vi "Load one I16bit Image with metadata from Tiff Stack file.vi"(7 "path to TIFF file":path=path "/HD1/Users/herbertlooser/Desktop/LadungssprŸher.tif", 8 "error in":errorcluster, 10 "Index of image\n to read":i32, 11 "I16 Image":T1) -> (0 "error out":errorcluster, 3 "I16 Image dup":T1)   [LabVIEW 2013, in "Tiff reader.lvlib"]
doc: "This .vi is taken from an online tiff reader. It is able to read 32-bit floating point .tiff images."
uses:
  Tiff reader.lvlib
  <vilib>/vision/Image Controls.llb/IMAQ Image.ctl
panel:
  out "Custom Data":string[](array[string])
  out "Keys":string[](array[string])
  out "I16":i16[][](array[numeric])
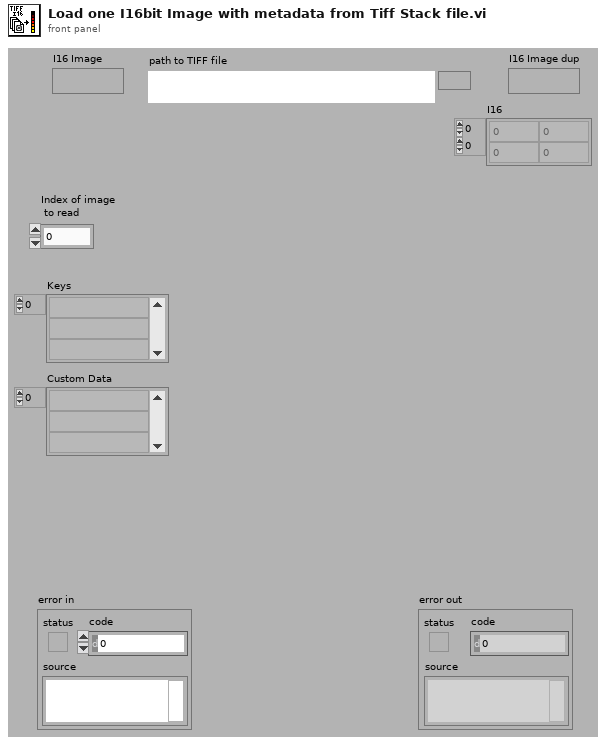
[diagram p1: front panel]
types:
  T1 = typedef "IMAQ Image.ctl" = refnum<image>
  T2 = enum16{"open", "replace", "create", "open or create", "replace or create", "replace or create with confirmation"}
  T3 = typedef "Tiff reader.lvlib/IFD Entry.ctl" = cluster{"Tag":u16, "Type":T4, "Count":u32, "Val/Offs":u32, "Is Pointer?":bool, "Byte stream index":i32}
  T4 = typedef "Tiff reader.lvlib/FieldTypes.ctl" = enum16{"NULL", "U8", "ASCII7", "U16", "U32", "RATIONAL", "SByte(I8)", "Undef(8Bit)", "I16", "I32", "SRat(4B:4B)", "SGL(4Byte)", "DBL(8Byte)"}
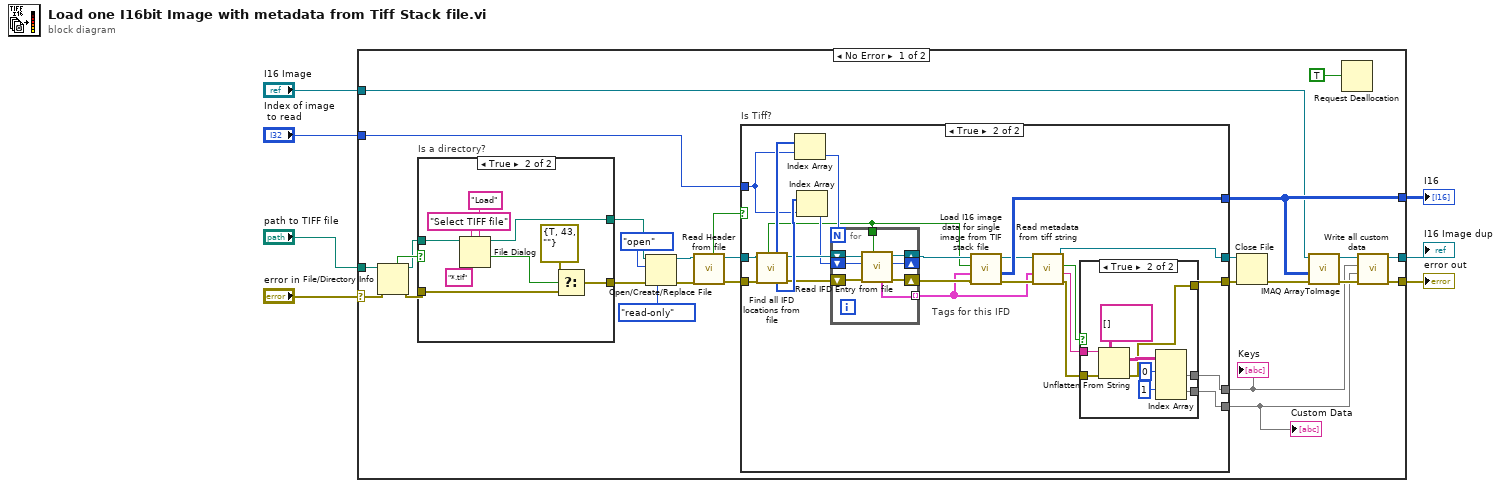
[diagram p0: block diagram]
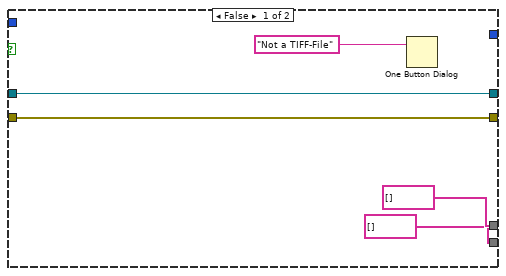
[diagram p2: hidden frame]
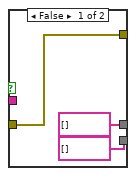
[diagram p3: hidden frame]
diagram:
  n1 = case shown="No Error" "error in" {
    selector: "error in" -> [w11 w95]
    tunnel: "path to TIFF file" -> [w33 _]
    tunnel: "Index of image\n to read" -> [w21 _]
    tunnel: [w19 _] -> w5
    tunnel: [w15 w94] -> w4
    tunnel: [w14 w95] -> w3
    tunnel: "I16 Image" -> [w10 w94]
    frame No Error {
      n2 = File/Directory Info(path=w33, error in=w11) -> (path out=w8:path, directory=w34:bool, error out=w32:errorcluster)  [unwired: 4 out]
      n3 = case "Is a directory?" shown="True" w34 {
        tunnel: w32 -> [w84 w90]
        tunnel: w8 -> [w83 w89]
        tunnel: [w84 w85] -> w24
        tunnel: [w83 w86] -> w23
        frame False {
        }
        frame True {
          n4 = File Dialog(5:"Load" ("button label"), 6:"*.tif" ("pattern"), 7:"Select TIFF file" ("prompt"), 11:w89) -> (1:w91:bool, 3:w86:path)  [unwired: 1 in, 4 out]
          n5 = Select(t=errorcluster {"status"=TRUE, "code"=43, "source"=""} ("error in (no error)"), s=w91, f=w90) -> (s? t:f=w85:errorcluster)
        }
      }
      n6 = Open/Create/Replace File(file path (use dialog)=w23, error in=w24, operation (0:open)=T2."open", access (0:read/write)=enum16{"read/write", "read-only", "write-only"}."read-only") -> (refnum out=w22:refnum<file>, error out=w25:errorcluster)  [unwired: 3 out]
      n7 = call "Read Header from file.vi"("error in"=w25, "File"=w22) -> ("error out"=w29:errorcluster, "File"=w28:refnum<file>, "isTIFF"=w30:bool)  [unwired: 5 out]
      n8 = case "Is Tiff?" shown="True" w30 {
        tunnel: w29 -> [w37 w51]
        tunnel: w28 -> [w38 w52]
        tunnel: [_ w62] -> w19
        tunnel: [w37 w53] -> w18
        tunnel: [w38 w59] -> w17
        tunnel: w21 -> [_ w40]
        tunnel: [string[] [] w56] -> w12
        tunnel: [string[] [] w55] -> w9
        frame False {
          n9 = One Button Dialog(message="Not a TIFF-File") -> ()  [unwired: 2 out]
        }
        frame True {
          # "Tags for this IFD"
          n10 = call "Find all IFD locations from file.vi"("error in"=w51, "File"=w52) -> ("error out"=w47:errorcluster, "File"=w49:refnum<file>, "1st tag locations"=w50:u32[], "# of tags in each IFD"=w44:u16[], "Litt/BigEnd"=w42:bool)  [unwired: 5 out]
          n11 = Index Array(array=w44, index=w40) -> (element=w43:u16)
          n12 = Index Array(array=w50, index=w40) -> (element=w48:u32)
          n13 = for {
            N: w43 -> [_]
            shift-right: [w66] -> w45
            shift-left: w49 -> [w70]
            shift-right: [w67] -> _
            shift-left: w48 -> [w63]
            tunnel: [w64] -> w41 mode=indexing
            tunnel: w42 -> [w65]
            shift-right: [w68] -> w46
            shift-left: w47 -> [w69]
            n14 = call "Read IFD Entry from file.vi"("Litt/BigEnd"=w65, "error in"=w69, "Tag location in"=w63, "File"=w70) -> ("error out"=w68:errorcluster, "Next Tag location Out\n(IN + 12)"=w67:i64, "File"=w66:refnum<file>, "Tag"=w64:T3)  [unwired: 1 in, 3 out]
          }
          n15 = call "Load I16 image data for single image from TIF stack file.vi"("error in"=w46, "DirEntries"=w41, "Litt/BigEnd"=w42, "File"=w45) -> ("error out"=w60:errorcluster, "Gray16"=w62:i16[][], "File"=w61:refnum<file>)  [unwired: 5 out]
          n16 = call "Read metadata from tiff string.vi"("error in"=w60, "DirEntries"=w41, "Tiff image stack"=w61) -> ("error out"=w57:errorcluster, "Metadata string"=w58:string, "Tag exists?"=w54:bool, "Tiff image stack dup"=w59:refnum<file>)  [unwired: 1 in, 4 out]
          n17 = case shown="True" w54 {
            tunnel: w58 -> [_ w82]
            tunnel: w57 -> [w73 w80]
            tunnel: [string[] [] w78] -> w56
            tunnel: [string[] [] w77] -> w55
            tunnel: [w73 w74] -> w53
            frame False {
            }
            frame True {
              n18 = Unflatten From String(type=string[][] [], binary string=w82, error in (no error)=w80) -> (value=w79:string[][], error out=w74:errorcluster)  [unwired: 3 out]
              n19 = Index Array(array=w79, index (row) #1=0 ("index (row)"), index (row) #2=1 ("index (row)")) -> (element #1=w78:string[], element #2=w77:string[])  [unwired: 2 in]
            }
          }
        }
      }
      "Keys" <- w12
      "Custom Data" <- w9
      n20 = Close File(refnum=w17, error in=w18) -> (error out=w20:errorcluster)  [unwired: 1 out]
      n21 = call "IMAQ ArrayToImage"("error in (no error)"=w20, "Image Pixels (I16)"=w19, "Image"=w10) -> ("error out"=w13:errorcluster, "Image Out"=w16:T1)  [unwired: 3 in, 4 out]
      n22 = Request Deallocation(TRUE ("flag")) -> ()
      n23 = call "Write all custom data.vi"("error in (no error)"=w13, "Custom Data"=w9, "Keys"=w12, "img"=w16) -> ("error out"=w14:errorcluster, "Image (duplicate)"=w15:T1)  [unwired: 6 out]
    }
    frame Error {
    }
  }
  "error out" <- w3
  "I16" <- w5
  "I16 Image dup" <- w4
